vi "Exmaple_DictionaryClass.vi"() -> ()   [LabVIEW 2013]
uses:
  DictionaryClass/Dictionary.lvclass
  DictionaryStringClass/DictionaryString.lvclass
  DictionaryClass/Dictionary.lvclass/Dictionary.ctl
panel:
  out "error out 2":errorcluster caption="Fehler (Ausgang)"
  out "Value":string
  out "Dict":variant
  out "Wert":variant
  out "error out":errorcluster caption="Fehler (Ausgang)"
  in  "error in (no error)":errorcluster caption="Fehler (Eingang, kein Fehler)"
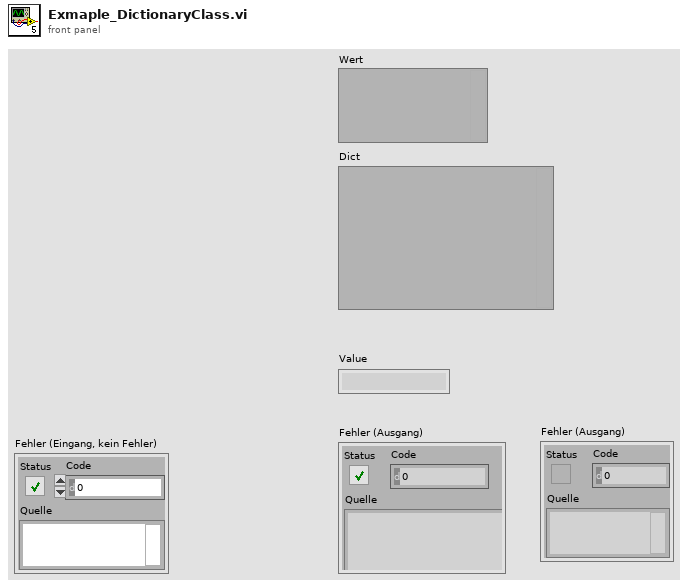
[diagram p1: front panel]
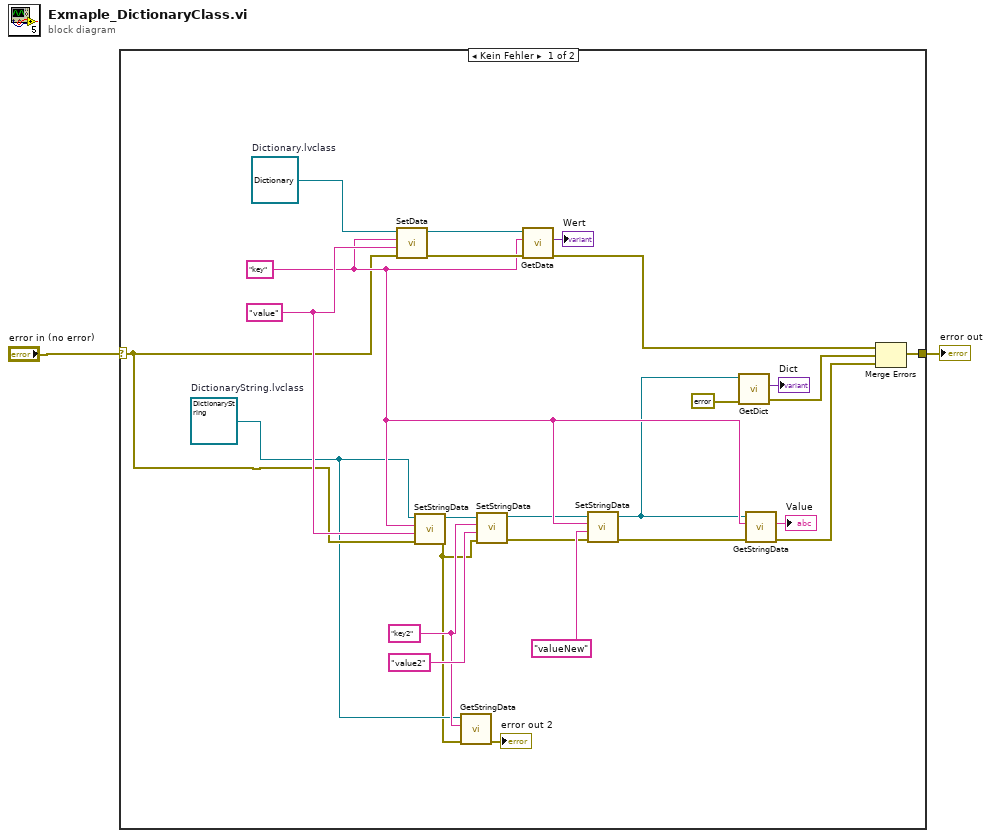
[diagram p0: block diagram]
diagram:
  n1 = case shown="Kein Fehler" "error in (no error)" {
    selector: "error in (no error)" -> [w7 w28]
    tunnel: [w22 w28] -> w1
    frame No Error {
      w6 = refnum<class "DictionaryString.lvclass"> refnum  # DictionaryString.lvclass
      w8 = "key2" ("Name")
      w24 = "value" ("Name")
      w19 = "key" ("Name")
      w20 = refnum<class "Dictionary.lvclass"> refnum  # Dictionary.lvclass
      n2 = call-dynamic "SetData.vi"("error in (no error)"=w7, "Data"=w24, "Key"=w19, "Dictionary Eingang"=w20) -> ("error out"=w26:errorcluster, "Dictionary Ausgang"=w4:refnum<class "Dictionary.lvclass">)  [unwired: 6 in]
      n3 = call-dynamic "SetStringData.vi"("error in (no error)"=w7, "Value"=w24, "Name"=w19, "DictionaryString Eingang"=w6) -> ("error out"=w5:errorcluster, "DictionaryString Ausgang"=w13:refnum<class "DictionaryString.lvclass">)  [unwired: 6 in]
      n4 = call-dynamic "GetStringData.vi"("error in (no error)"=w5, "Name"=w8, "DictionaryString Eingang"=w6) -> ("error out"=→"error out 2":errorcluster)  [unwired: 6 in, 2 out]
      n5 = call-dynamic "SetStringData.vi"("error in (no error)"=w5, "Value"="value2", "Name"=w8, "DictionaryString Eingang"=w13) -> ("error out"=w12:errorcluster, "DictionaryString Ausgang"=w11:refnum<class "DictionaryString.lvclass">)  [unwired: 6 in]
      n6 = call-dynamic "GetData.vi"("error in (no error)"=w26, "Name"=w19, "Dictionary Eingang"=w4) -> ("error out"=w21:errorcluster, "Wert"=→"Wert":variant)  [unwired: 6 in, 1 out]
      n7 = call-dynamic "SetStringData.vi"("error in (no error)"=w12, "Value"="valueNew", "Name"=w19, "DictionaryString Eingang"=w11) -> ("error out"=w16:errorcluster, "DictionaryString Ausgang"=w17:refnum<class "DictionaryString.lvclass">)  [unwired: 6 in]
      n8 = call "GetDict.vi"("error in (no error)"=errorcluster {"status"=FALSE, "code"=0, "source"=""}, "Dictionary (Eingang)"=w17) -> ("error out"=w15:errorcluster, "Dict"=→"Dict":variant)  [unwired: 7 in, 1 out]
      n9 = call-dynamic "GetStringData.vi"("error in (no error)"=w16, "Name"=w19, "DictionaryString Eingang"=w17) -> ("error out"=w14:errorcluster, "Value"=→"Value":string)  [unwired: 6 in, 1 out]
      n10 = Merge Errors(w21, w15, w14) -> (w22:errorcluster)
    }
    frame Error {
    }
  }
  "error out" <- w1
